vi "getModeByName.vi"(8 "error in (no error)":errorcluster, 10 "device_name":string, 11 "deviceDataBase in":refnum<class "deviceDataBase.lvclass">) -> (0 "error out":errorcluster, 2 "mode":enum16{"current", "voltage"}[](array[ring]), 3 "deviceDataBase out":refnum<class "deviceDataBase.lvclass">)   [LabVIEW 2011, in "Tools.lvlib" / "DatabaseHelpers.lvlib" / "deviceDataBase.lvclass"]
uses:
  deviceDataBase.lvclass
  deviceDataBase.lvclass/deviceDataBase.ctl
  Database Objects/device/device.lvclass
  Database Objects/device/EthernetSupply/ethernetSupply.lvclass
  Database Objects/DeviceArray/DeviceArray.lvclass
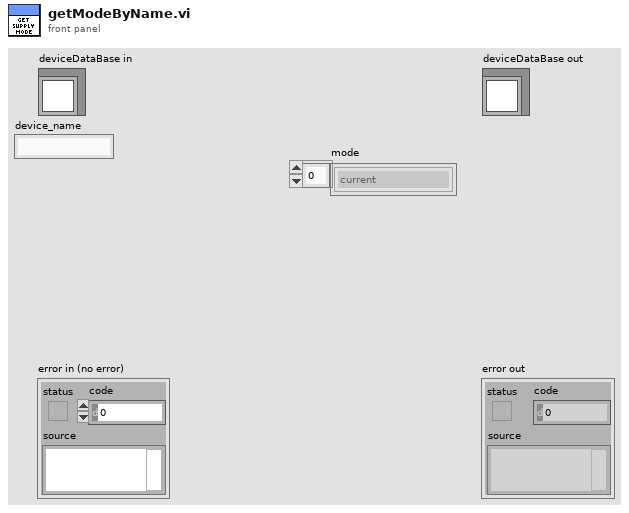
[diagram p1: front panel]
types:
  T1 = enum16{"digitalOutput", "digitalInput", "analogOutput", "analogInput", "rfOutput", "ethernetSupply"}
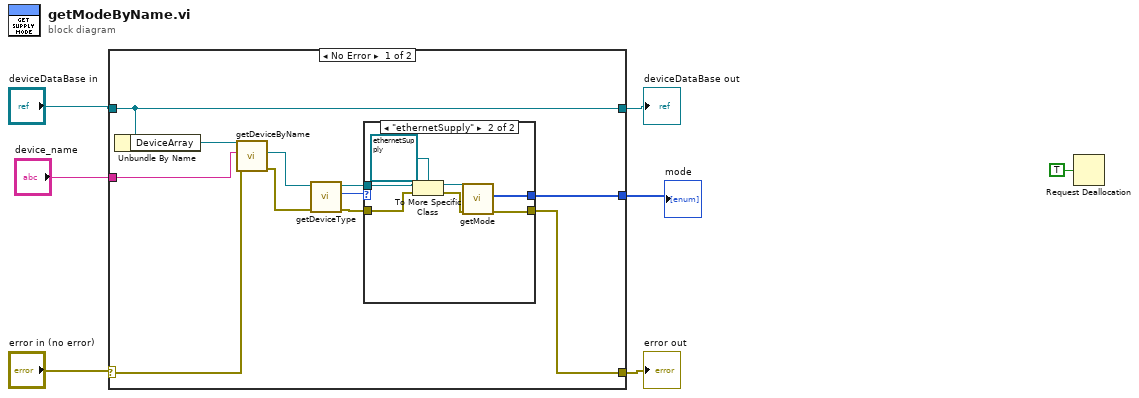
[diagram p0: block diagram]
diagram:
  n1 = case shown="No Error" "error in (no error)" {
    selector: "error in (no error)" -> [w15 w28]
    tunnel: [w9 w28] -> w5
    tunnel: [w18 w27] -> w4
    tunnel: "deviceDataBase in" -> [w18 w27]
    tunnel: "device_name" -> [w16 _]
    tunnel: [w8 _] -> w1
    frame No Error {
      n2 = Unbundle By Name(w18) -> ("DeviceArray"=w17:refnum<class "DeviceArray.lvclass">)
      n3 = call "getDeviceByName.vi"("error in (no error)"=w15, "deviceName"=w16, "DeviceArray in"=w17) -> ("error out"=w13:errorcluster, "device.lvclass"=w14:refnum<class "device.lvclass">)  [unwired: 5 in, 2 out]
      n4 = call-dynamic "getDeviceType.vi"("error in (no error)"=w13, "device.lvclass in"=w14) -> ("error out"=w10:errorcluster, "type"=w12:T1, "device.lvclass out"=w11:refnum<class "device.lvclass">)  [unwired: 7 in]
      n5 = case shown="\"ethernetSupply\"" w12 {
        tunnel: w11 -> [_ w26]
        tunnel: w10 -> [w19 w25]
        tunnel: [w19 w20] -> w9
        tunnel: [_ w21] -> w8
        frame Default {
        }
        frame "ethernetSupply" {
          n6 = To More Specific Class(target class=refnum<class "ethernetSupply.lvclass"> refnum ("Tools.lvlib:DatabaseHelpers.lvlib:EthernetSupply.lvclass"), reference=w26, error in=w25) -> (specific class reference=w23:refnum<class "ethernetSupply.lvclass">, error out=w22:errorcluster)
          n7 = call "getMode.vi"("error in (no error)"=w22, "ethernetSupply in"=w23) -> ("error out"=w20:errorcluster, "mode"=w21:enum16{"current", "voltage"}[])  [unwired: 7 in, 1 out]
        }
      }
    }
    frame Error {
    }
  }
  "error out" <- w5
  "deviceDataBase out" <- w4
  "mode" <- w1
  n8 = Request Deallocation(TRUE ("flag")) -> ()
